vi "matrici_v0_v34.vi"() -> ()   [LabVIEW 2009]
panel:
  in  "stop":bool
  in  "Coloana":u8(slide)=2 scale=0.0..4.0
  out "Coloana selectata":bool[](array[boolean])=[FALSE, FALSE, TRUE, FALSE, FALSE, TRUE, TRUE]
  in  "Array":bool[][](array[boolean])=[[TRUE, FALSE, FALSE, FALSE, TRUE], [FALSE, TRUE, FALSE, FALSE, FALSE], [FALSE, FALSE, TRUE, FALSE, FALSE], [FALSE, TRUE, FALSE, FALSE, FALSE], [TRUE, FALSE, FALSE, TRUE, FALSE], [FALSE, FALSE, TRUE, TRUE, FALSE], [TRUE, FALSE, TRUE, TRUE, FALSE]]
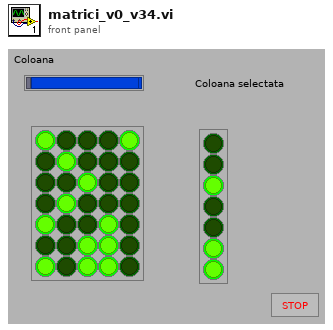
[diagram p1: front panel]
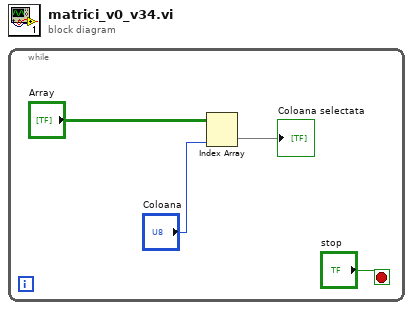
[diagram p0: block diagram]
diagram:
  n1 = while {
    stop <- "stop" stop-if-true
    n2 = Index Array(array="Array", index (col)="Coloana") -> (element=→"Coloana selectata":bool[])  [unwired: 1 in]
  }
